vi "SEND PUBREC.vi"(8 "error in (no error)":errorcluster, 10 "Message ID":u16=10 format="%x", 11 "connection ID":refnum<k5>) -> (0 "error out":errorcluster, 3 "connection ID out":refnum<k5>)   [LabVIEW 2020, in "DAQIO MQTT.lvlib"]
uses:
  DAQIO MQTT.lvlib
  Controls/MessageType.ctl
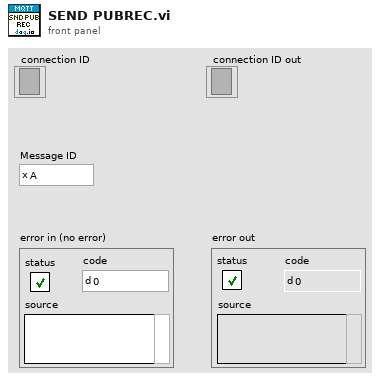
[diagram p1: front panel]
types:
  T1 = typedef "DAQIO MQTT.lvlib/MessageType.ctl" = enum32{"Reserved", "CONNECT", "CONNACK", "PUBLISH", "PUBACK", "PUBREC", "PUBREL", "PUBCOMP", "SUBSCRIBE", "SUBACK", "UNSUBSCRIBE", "UNSUBACK", "PINGREQ", "PINGRESP", "DISCONNECT", "Reserved2"}
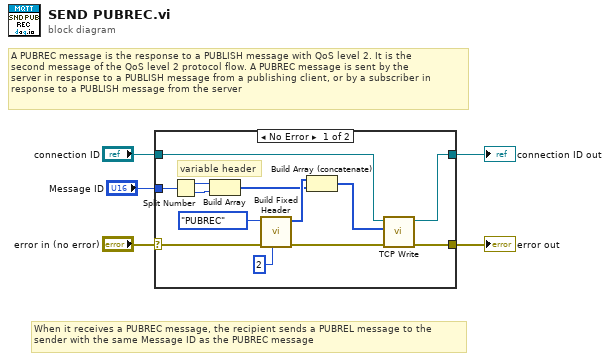
[diagram p0: block diagram]
diagram:
  # "When it receives a PUBREC message, the recipient sends a PUBREL message to the\nsender with the same Message ID as the PUBREC message"
  # "A PUBREC message is the response to a PUBLISH message with QoS level 2. It is the\nsecond message of the QoS level 2 protocol flow. A PUBREC message is sent by the\nserver in response to a PUBLISH message from a publishing client, or by a subscriber in\nresponse to a PUBLISH message from the server"
  n1 = case shown="No Error" "error in (no error)" {
    selector: "error in (no error)" -> [w13 w20]
    tunnel: [w9 w20] -> w4
    tunnel: "connection ID" -> [w8 w19]
    tunnel: [w7 w19] -> w2
    tunnel: "Message ID" -> [w6 _]
    frame No Error {
      # "variable header"
      n2 = Split Number(x=w6) -> (hi(x)=w16:u8, lo(x)=w15:u8)
      n3 = Build Array(w16, w15) -> (w12:u8[])
      n4 = call "Build Fixed Header.vi"("Remaining Length"=u32 2, "error in (no error)"=w13, "MessageType"=MessageType."PUBREC") -> ("error out"=w10:errorcluster, "Fixed Header"=w17:u8[])  [unwired: 7 in]
      n5 = Build Array (concatenate)(w17, w12) -> (w11:u8[])
      n6 = call "TCP Write.vi"("error in (no error)"=w10, "data in"=w11, "connection ID"=w8) -> ("error out"=w9:errorcluster, "connection ID out"=w7:refnum<k5>)  [unwired: 6 in, 1 out]
    }
    frame Error {
    }
  }
  "error out" <- w4
  "connection ID out" <- w2
